vi "Loop_SM.vi"() -> ()   [LabVIEW 2017, in "LED Signal.lvlib"]
uses:
  LED Signal.lvlib
  <vilib>/Rock Robotics/WPI/SerialPort/WPI_SerialPort.ctl
  TypeDefs/ENUM_LED_Drive_Mode.ctl
  ENUM_State.ctl
  ENUM_Action.ctl
  Cluster_SM to HW Data.ctl
  ENUM_HW LED Commands.ctl
  Globals/Global_STOP.vi
  Global_SM_Data Out.vi
panel:
  in  "Drive Mode":T1
  in  "Select Serial Port":T2
  in  "Vision On Target":bool
  in  "Hopper Empty":bool
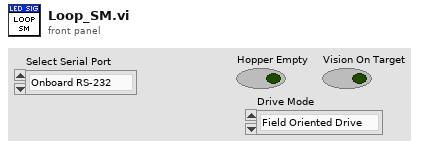
[diagram p1: front panel]
types:
  T1 = typedef "LED Signal.lvlib/ENUM_LED_Drive_Mode.ctl" = enum16{"Field Oriented Drive", "Angled Drive", "Normal Drive"}
  T2 = typedef "WPI_SerialPort.ctl" = enum16{"Onboard RS-232", "MXP TTL", "USB 1", "USB 2"}
  T3 = typedef "LED Signal.lvlib/Cluster_SM to HW Data.ctl" = cluster{"Serial Port":T2, "Cmd List":T4[]}
  T4 = typedef "LED Signal.lvlib/ENUM_HW LED Commands.ctl" = enum16{"No  Command", "Angled Drive; A", "Field Oriented Drive; D", "Normal Drive; d", "Camera Lined Up; C", "Camera Misallined; c", "Balls in Hopper; B", "Hopper Empty; b"}
  T5 = typedef "LED Signal.lvlib/ENUM_Action.ctl" = enum16{"No Action", "Reset Time", "Reset All", "Set Camera Status", "Set Hopper Status", "Set Drive Mode", "Clear Commands"}
  T6 = typedef "LED Signal.lvlib/ENUM_State.ctl" = enum16{"Startup", "Idle", "Shutdown", "Monitoring"}
  T7 = cluster{"Actions":T5[], "State":T6, "Current Time":timestamp, "Start Time":timestamp, "Loop Time (ms)":u32, "SM LED_HW Cmd Data":T3, "Hopper Empty":bool, "Drive Mode":T1, "Vision On Target":bool}
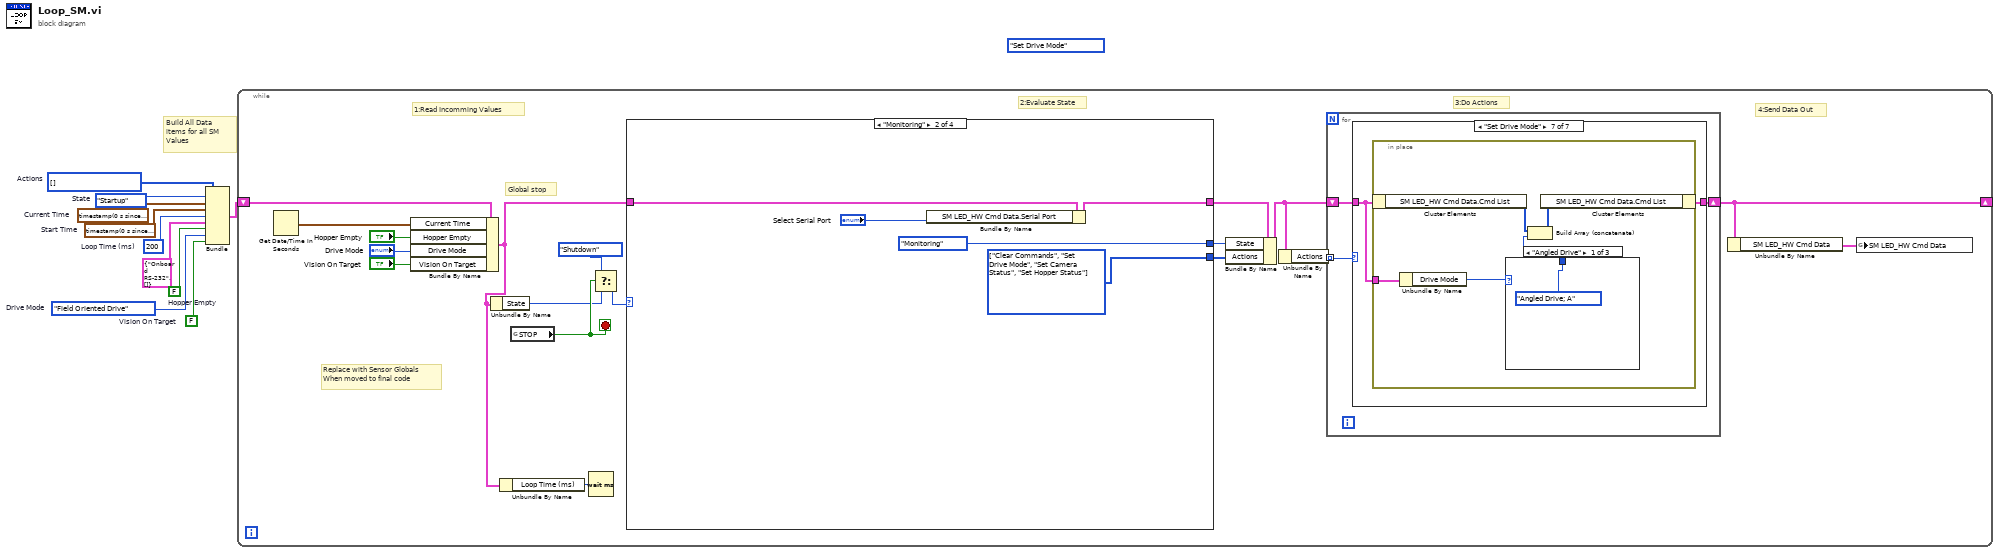
[diagram p0: block diagram]
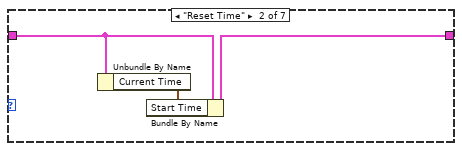
[diagram p3: hidden frame]
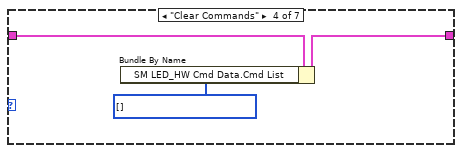
[diagram p5: hidden frame]
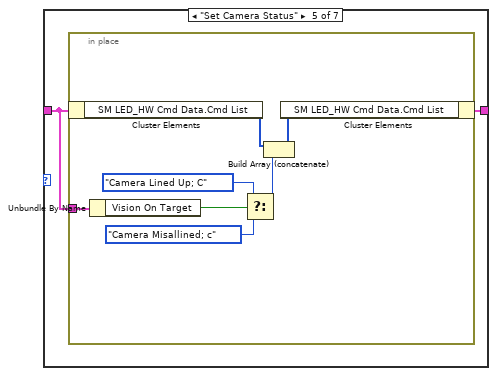
[diagram p6: hidden frame]
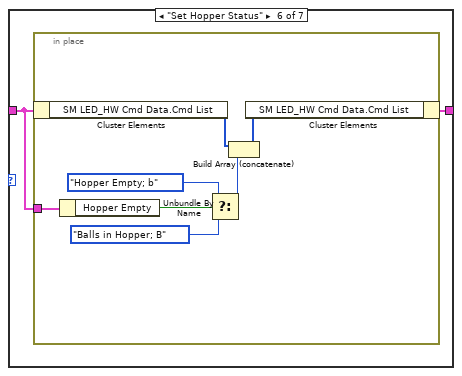
[diagram p7: hidden frame]
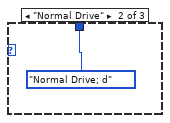
[diagram p8: hidden frame]
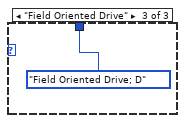
[diagram p9: hidden frame]
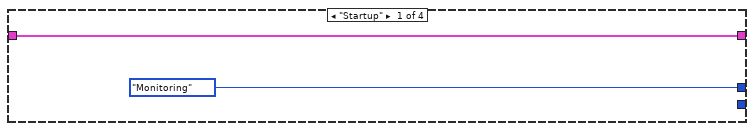
[diagram p10: hidden frame]
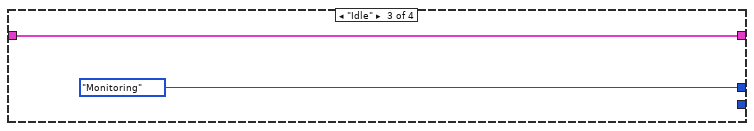
[diagram p11: hidden frame]
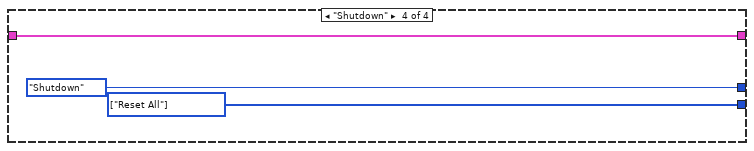
[diagram p12: hidden frame]
diagram:
  w3 = ENUM_LED_Drive_Mode."Field Oriented Drive"  # Drive Mode
  (unwired) ENUM_Action."Set Drive Mode" ("Action")
  w4 = FALSE  # Vision On Target
  w5 = FALSE  # Hopper Empty
  w6 = u32 200  # Loop Time (ms)
  w7 = T5[] [] items=["No Action", "Reset Time", "Reset All", "Set Camera Status", "Set Hopper Status", "Set Drive Mode", "Clear Commands"]  # Actions
  w8 = timestamp(0 s since 1904-01-01)  # Start Time
  w9 = timestamp(0 s since 1904-01-01)  # Current Time
  w10 = ENUM_State."Startup"  # State
  # "Build All Data items for all SM Values"
  n1 = Bundle("Actions"=w7, "State"=w10, "Current Time"=w9, "Start Time"=w8, "Loop Time (ms)"=w6, "SM LED_HW Cmd Data"=T3 {"Serial Port"=enum."Onboard RS-232", "Cmd List"=[]}, "Hopper Empty"=w5, "Drive Mode"=w3, "Vision On Target"=w4) -> (w2:T7)  [unwired: 1 in]
  n2 = while {
    shift-right: [w17] -> _
    shift-left: w2 -> [w27]
    stop <- w21 stop-if-true
    # "Replace with Sensor Globals\nWhen moved to final code"
    # "1:Read Incomming Values"
    # "2:Evaluate State"
    # "3:Do Actions"
    # "4:Send Data Out"
    # "Global stop"
    n3 = Get Date/Time In Seconds() -> (seconds since 1Jan1904=w26:timestamp)
    n4 = Bundle By Name(cluster=w27, "Current Time"=w26, "Hopper Empty"="Hopper Empty", "Drive Mode"="Drive Mode", "Vision On Target"="Vision On Target") -> (w16:T7)
    n5 = Unbundle By Name(w16) -> ("State"=w19:T6)
    n6 = Unbundle By Name(w16) -> ("Loop Time (ms)"=w11:u32)
    n7 = global read "Global_STOP.vi" "STOP"() -> (w21:bool)
    n8 = Wait (ms)(milliseconds to wait=w11) -> ()  [unwired: 1 out]
    n9 = Select(t=ENUM_State."Shutdown" ("State"), s=w21, f=w19) -> (s? t:f=w18:T6)
    n10 = case shown="\"Monitoring\"" w18 {
      tunnel: w16 -> [w69 w72 w76 w79]
      tunnel: [w69 w71 w76 w79] -> w24
      tunnel: [ENUM_State."Monitoring" ("State") ENUM_State."Monitoring" ("State") ENUM_State."Monitoring" ("State") ENUM_State."Shutdown" ("State")] -> w23
      tunnel: [_ w73 _ w77] -> w22
      frame "Startup" {
      }
      frame "Monitoring" {
        w73 = T5[] [enum."Clear Commands", enum."Set Drive Mode", enum."Set Camera Status", enum."Set Hopper Status"] items=["No Action", "Reset Time", "Reset All", "Set Camera Status", "Set Hopper Status", "Set Drive Mode", "Clear Commands"] ("Actions")
        n11 = Bundle By Name(cluster=w72, "SM LED_HW Cmd Data.Serial Port"="Select Serial Port") -> (w71:T7)
      }
      frame "Idle" {
      }
      frame "Shutdown" {
        w77 = T5[] [enum."Reset All"] items=["No Action", "Reset Time", "Reset All", "Set Camera Status", "Set Hopper Status", "Set Drive Mode", "Clear Commands"] ("Actions")
      }
    }
    n12 = Bundle By Name(cluster=w24, "State"=w23, "Actions"=w22) -> (w25:T7)
    n13 = Unbundle By Name(w25) -> ("Actions"=w28:T5[])
    n14 = for {
      tunnel: w28 -> [w29] mode=indexing
      shift-right: [w31] -> w17
      shift-left: w25 -> [w30]
      n15 = case shown="\"Set Drive Mode\"" w29 {
        tunnel: w30 -> [w32 w35 w36 w39 w40 w49 w58]
        tunnel: [w32 w34 w36 w38 w41 w50 w59] -> w31
        frame "No Action" {
        }
        frame "Reset Time" {
          n16 = Unbundle By Name(w35) -> ("Current Time"=w33:timestamp)
          n17 = Bundle By Name(cluster=w35, "Start Time"=w33) -> (w34:T7)
        }
        frame "Reset All" {
        }
        frame "Clear Commands" {
          w37 = T4[] [] items=["No  Command", "Angled Drive; A", "Field Oriented Drive; D", "Normal Drive; d", "Camera Lined Up; C", "Camera Misallined; c", "Balls in Hopper; B", "Hopper Empty; b"] ("SM LED_HW Cmd OUT.Cmd List")
          n18 = Bundle By Name(cluster=w39, "SM LED_HW Cmd Data.Cmd List"=w37) -> (w38:T7)
        }
        frame "Set Camera Status" {
          n19 = in-place {
            in-place-border: w40 -> [w48]
            n20 = in-place-cluster #1(w40) -> ("SM LED_HW Cmd Data.Cmd List"=w42:T4[])
            n21 = Unbundle By Name(w48) -> ("Vision On Target"=w43:bool)
            n22 = Select(t=ENUM_HW_LED_Commands."Camera Lined Up; C" ("Cmd"), s=w43, f=ENUM_HW_LED_Commands."Camera Misallined; c" ("Cmd")) -> (s? t:f=w45:T4)
            n23 = Build Array (concatenate)(w42, w45) -> (w44:T4[])
            n24 = in-place-cluster #1("SM LED_HW Cmd Data.Cmd List"=w44) -> (w41:T7)
          }
        }
        frame "Set Hopper Status" {
          n25 = in-place {
            in-place-border: w49 -> [w57]
            n26 = in-place-cluster #2(w49) -> ("SM LED_HW Cmd Data.Cmd List"=w51:T4[])
            n27 = Unbundle By Name(w57) -> ("Hopper Empty"=w52:bool)
            n28 = Select(t=ENUM_HW_LED_Commands."Hopper Empty; b" ("Cmd"), s=w52, f=ENUM_HW_LED_Commands."Balls in Hopper; B" ("Cmd")) -> (s? t:f=w54:T4)
            n29 = Build Array (concatenate)(w51, w54) -> (w53:T4[])
            n30 = in-place-cluster #2("SM LED_HW Cmd Data.Cmd List"=w53) -> (w50:T7)
          }
        }
        frame "Set Drive Mode" {
          n31 = in-place {
            in-place-border: w58 -> [w64]
            n32 = in-place-cluster #3(w58) -> ("SM LED_HW Cmd Data.Cmd List"=w60:T4[])
            n33 = Unbundle By Name(w64) -> ("Drive Mode"=w62:T1)
            n34 = case shown="\"Angled Drive\"" w62 {
              tunnel: [ENUM_HW_LED_Commands."Angled Drive; A" ("Cmd") ENUM_HW_LED_Commands."Normal Drive; d" ("Cmd") ENUM_HW_LED_Commands."Field Oriented Drive; D" ("Cmd")] -> w61
              frame "Angled Drive" {
              }
              frame "Normal Drive" {
              }
              frame "Field Oriented Drive" {
              }
            }
            n35 = Build Array (concatenate)(w60, w61) -> (w63:T4[])
            n36 = in-place-cluster #3("SM LED_HW Cmd Data.Cmd List"=w63) -> (w59:T7)
          }
        }
      }
    }
    n37 = Unbundle By Name(w17) -> ("SM LED_HW Cmd Data"=w12:T3)
    n38 = global write "Global_SM_Data Out.vi" "SM LED_HW Cmd Data"(w12) -> ()
  }
